vi "Trap_Write_Wfm.vi"(8 "error in (no error)":errorcluster caption="entrée d'erreur (pas d'erreur)", 11 "SOFTWARE Inputs":T1={"Application Directory"=path "D:/S.O.F.T.S/LABVIEW/PIL", "Software Version"="1.0.0", "Data Path"=path "D:/PIRENEA/DATA", "XML Path"=path "D:/PIRENEA/DATA", "XML File Filter"="*.xml", "XML Saved Path"=path "D:/S.O.F.T.S/LABVIEW/PIL/resources", "Excit Scripts Path"=path "D:/PIRENEA/EXCIT_SCRIPTS", "Excit Scripts File Filter"="*.txt", "Excit Waveforms Path"=path "D:/PIRENEA/EXCIT_WFMS", "Excit Waveforms File Filter"="*.bin", "Timing Scripts Path"=path "D:/PIRENEA/TIMING_SCRIPTS", "Timing Scripts File Filter"="*.txt", "Timing Waveforms Path"=path "D:/PIRENEA/TIMING_WFMS", "Timing Waveforms File Filter"="*.bin", "Trapping Waveforms Path"=path "D:/PIRENEA/TRAPPING_WFMS", "Trapping Waveforms File Filter"="*.bin"}) -> (0 "error out":errorcluster caption="sortie d'erreur", 2 "Data written":dbl[](graph), 3 "Filename created":string)   [LabVIEW 2018]
doc: "From a start and end value, generates an adiabatic waveform of 2000 values (double).\nWrites this waveform into a binary file, in a big-endian format.\nDisplays the written data.\nDefault Path for the generated file is D:\\PIRENEA\\TRAPPING_WFMS"
uses:
  controls/SOFTWARE_Inputs.ctl
panel:
  in  "Slope":dbl=5.0 format="%#_13g"
  in  "Nb of values":i32=2000
  in  "End value":dbl
  in  "Start value":dbl=5.0
  in  "Adiabatic Form":enum16{"None", "Ramp", "Double Ramp", "RC"}(ring)=enum."Ramp"
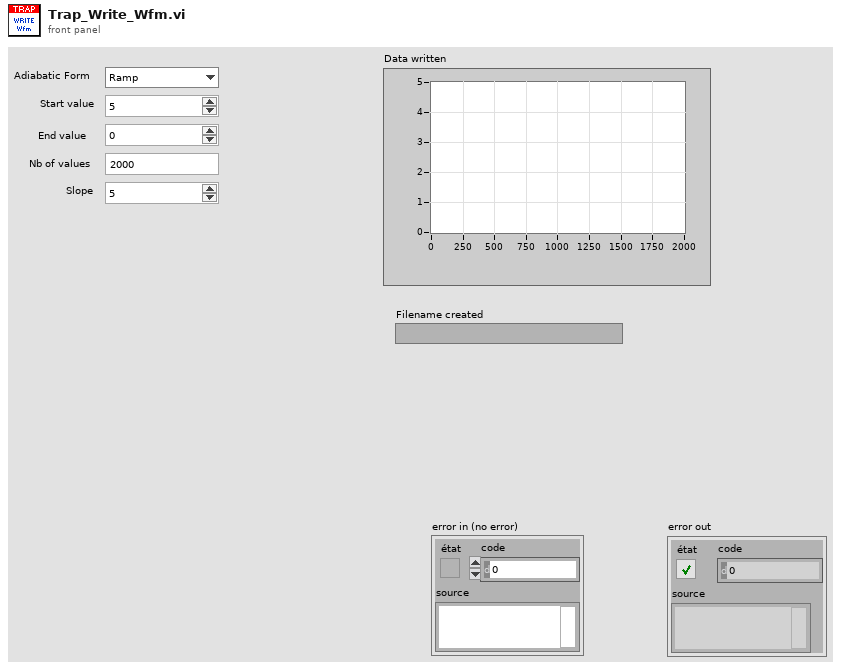
[diagram p1: front panel]
types:
  T1 = typedef "SOFTWARE_Inputs.ctl" = cluster{"Application Directory":path, "Software Version":string, "Data Path":path, "XML Path":path, "XML File Filter":string, "XML Saved Path":path, "Excit Scripts Path":path, "Excit Scripts File Filter":string, "Excit Waveforms Path":path, "Excit Waveforms File Filter":string, "Timing Scripts Path":path, "Timing Scripts File Filter":string, "Timing Waveforms Path":path, "Timing Waveforms File Filter":string, "Trapping Waveforms Path":path, "Trapping Waveforms File Filter":string}
  T2 = enum16{"open", "replace", "create", "open or create", "replace or create", "replace or create with confirmation"}
  T3 = enum16{"big-endian, network order", "native, host order", "little-endian"}
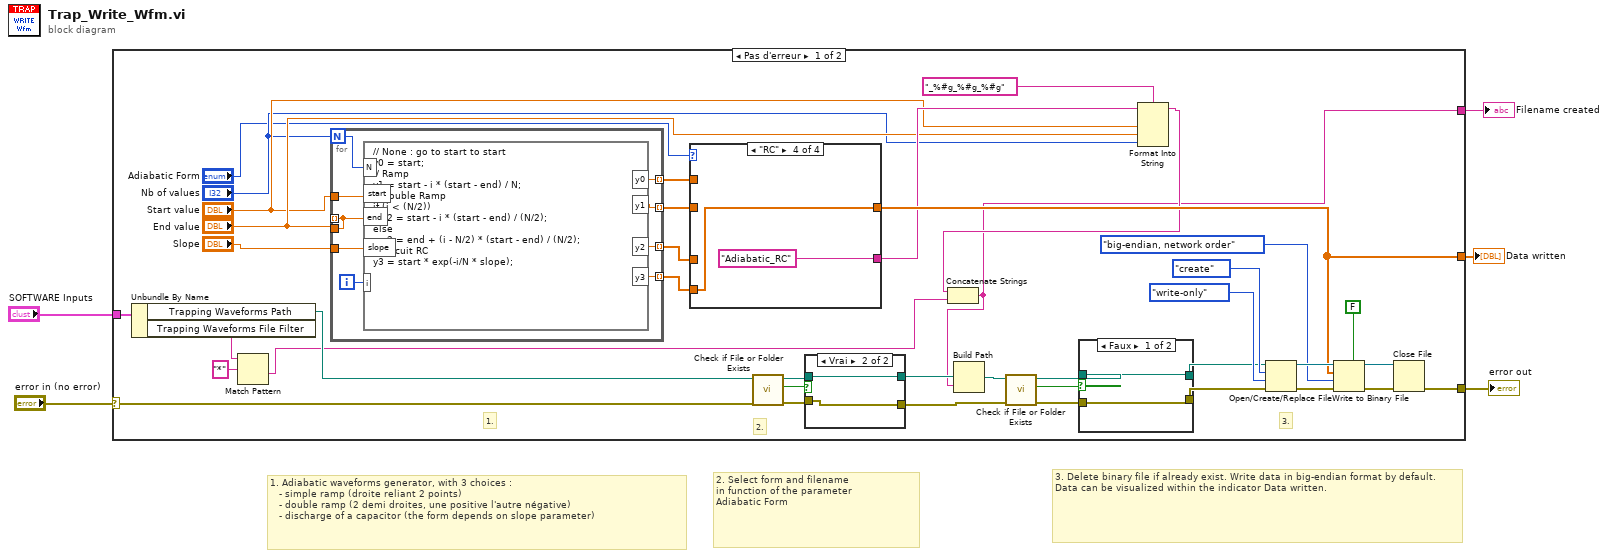
[diagram p0: block diagram]
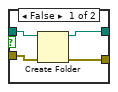
[diagram p2: hidden frame]
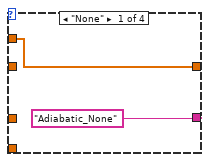
[diagram p3: hidden frame]
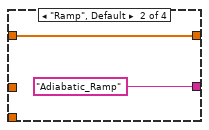
[diagram p4: hidden frame]
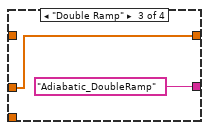
[diagram p5: hidden frame]
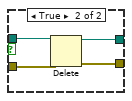
[diagram p6: hidden frame]
diagram:
  # "1. Adiabatic waveforms generator, with 3 choices :\n   - simple ramp (droite reliant 2 points)\n   - double ramp (2 demi droites, une positive l'autre négative)\n   - discharge of a capacitor (the form depends on slope parameter)"
  # "2. Select form and filename\nin function of the parameter\nAdiabatic Form"
  # "3. Delete binary file if already exist. Write data in big-endian format by default. Data can be visualized within the indicator Data written."
  n1 = case shown="Pas d'erreur" "error in (no error)" {
    selector: "error in (no error)" -> [w11 w75]
    tunnel: [w34 w75] -> w2
    tunnel: [w33 _] -> w5
    tunnel: "SOFTWARE Inputs" -> [w18 _]
    tunnel: [w6 _] -> w1
    frame No Error {
      # "3."
      # "2."
      # "1."
      n2 = Unbundle By Name(w18) -> ("Trapping Waveforms Path"=w17:path, "Trapping Waveforms File Filter"=w10:string)
      n3 = Match Pattern(string=w10, regular expression="*" ("expression régulière")) -> (after substring=w7:string)  [unwired: 1 in, 3 out]
      n4 = for {
        N: "Nb of values" -> [w67]
        tunnel: "Start value" -> [w66]
        tunnel: [w61] -> _ mode=indexing
        tunnel: [w65] -> w37 mode=indexing
        tunnel: [w64] -> w36 mode=indexing
        tunnel: [w63] -> w35 mode=indexing
        tunnel: "Slope" -> [w62]
        tunnel: "End value" -> [w61]
        tunnel: [w60] -> w32 mode=indexing
        i -> [w68]
        n5 = formula code="// None : go to start to start\ny0 = start;\n// Ramp\ny1 = start - i * (start - end) / N;\n// Double Ramp\nif (i < (N/2))\n   y2 = start - i * (start - end) / (N/2);\nelse\n   y2 = end + (i - N/2) * (start - end) / (N/2);\n// Circuit RC\ny3 = start * exp(-i/N * slope);"("start"=w66, "end"=w61, "i"=w68, "N"=w67, "slope"=w62) -> ("y1"=w65:dbl, "y2"=w64:dbl, "y3"=w63:dbl, "y0"=w60:dbl)
      }
      n6 = case shown="\"RC\"" "Adiabatic Form" {
        tunnel: w37 -> [_ w55 _ _]
        tunnel: w36 -> [_ _ w57 _]
        tunnel: w35 -> [_ _ _ w59]
        tunnel: [w52 w55 w57 w59] -> w33
        tunnel: ["Adiabatic_None" "Adiabatic_Ramp" "Adiabatic_DoubleRamp" "Adiabatic_RC"] -> w31
        tunnel: w32 -> [w52 _ _ _]
        frame "None" {
        }
        frame "Ramp", Default {
        }
        frame "Double Ramp" {
        }
        frame "RC" {
        }
      }
      n7 = call <vilib>:"Check if File or Folder Exists.vi"("error in (no error)"=w11, "path"=w17) -> ("error out"=w26:errorcluster, "file or folder exists?"=w29:bool, "dup path"=w28:path)  [unwired: 7 in]
      n8 = case shown="Vrai" w29 {
        tunnel: w28 -> [w49 w51]
        tunnel: [w48 w51] -> w27
        tunnel: w26 -> [w47 w50]
        tunnel: [w46 w50] -> w25
        frame False {
          n9 = Create Folder(path (use dialog)=w49, error in=w47) -> (created path=w48:path, error out=w46:errorcluster)  [unwired: 1 in, 1 out]
        }
        frame True {
        }
      }
      n10 = Format Into String(format string="_%#g_%#g_%#g", initial string=w31, "Start value", "End value", "Nb of values") -> (resulting string=w8:string)  [unwired: 1 in, 1 out]
      n11 = Concatenate Strings(w8, w7) -> (w6:string)
      n12 = Build Path(base path=w27, name or relative path=w6) -> (appended path=w24:path)
      n13 = call <vilib>:"Check if File or Folder Exists.vi"("error in (no error)"=w25, "path"=w24) -> ("error out"=w21:errorcluster, "file or folder exists?"=w22:bool, "dup path"=w23:path)  [unwired: 7 in]
      n14 = case shown="Faux" w22 {
        tunnel: w23 -> [w70 w74]
        tunnel: w21 -> [w69 w73]
        tunnel: [w70 w72] -> w19
        tunnel: [w69 w71] -> w20
        frame False {
        }
        frame True {
          n15 = Delete(path (use dialog)=w74, error in=w73) -> (deleted path=w72:path, error out=w71:errorcluster)  [unwired: 3 in, 1 out]
        }
      }
      n16 = Open/Create/Replace File(file path (use dialog)=w19, error in=w20, operation (0:open)=T2."create", access (0:read/write)=enum16{"read/write", "read-only", "write-only"}."write-only") -> (refnum out=w42:refnum<file>, error out=w43:errorcluster)  [unwired: 2 in, 1 out]
      n17 = Write to Binary File(file (use dialog)=w42, data=w33, error in=w43, 5:FALSE ("prepend array or string size? (T)"), 9:T3."big-endian, network order" ("byte order")) -> (refnum out=w45:refnum<file>, error out=w44:errorcluster)  [unwired: 1 in, 1 out]
      n18 = Close File(refnum=w45, error in=w44) -> (error out=w34:errorcluster)  [unwired: 1 out]
    }
    frame Error {
    }
  }
  "Data written" <- w5
  "Filename created" <- w1
  "error out" <- w2
